vi "Tutorial 08.vi"() -> ()   [LabVIEW 2014]
panel:
  out "Numeric":i32
  in  "stop":bool
  out "Random Number":dbl
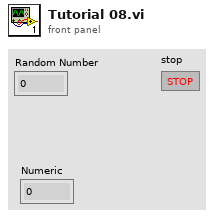
[diagram p1: front panel]
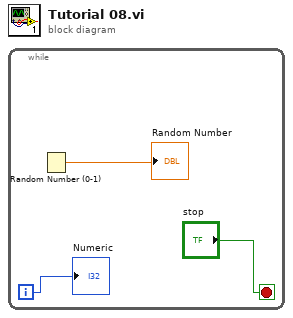
[diagram p0: block diagram]
diagram:
  n1 = while {
    i -> [w1]
    stop <- "stop" stop-if-true
    n2 = Random Number (0-1)() -> (number: 0 to 1=→"Random Number":dbl)
    "Numeric" <- w1
  }
